vi "Line Configuration Dialog.vi"(8 "error in":errorcluster, 9 "engine configuration in":refnum<class "engine configuration.lvclass">, 10 "tag bus configurable plugin module configuration":refnum<class "JSON_RPC_Interface configuration.lvclass">, 11 "Line":T3) -> (0 "error out":errorcluster, 1 "success":bool, 2 "changed":bool, 3 "Mappings out":T2)   [LabVIEW 2018, in "JSON_RPC_Interface editor node.lvclass"]
doc: "A dialog for allowing a user to specify the values of a new line."
uses:
  JSON_RPC_Interface editor node.lvclass
  module/configuration/Line.ctl
  <vilib>/NI/Tag Bus Module Framework/channel/TBM channel.lvclass
  C:/Program Files (x86)/National Instruments/LabVIEW 2018/vi.lib/NI/Tag Bus/tag/tag descriptor.lvclass
  Mappings.ctl
  Map.ctl
  permissions.ctl
  <vilib>/NI/Module Execution Interface/Engine Configuration/engine configuration.lvclass
  module/configuration/JSON_RPC_Interface configuration.lvclass
  C:/Program Files (x86)/National Instruments/LabVIEW 2018/vi.lib/NI/Configuration Framework/serializable configuration/NISE_CEF_serializable configuration.lvclass
  <vilib>/NI/Tag Bus/tag/tag descriptor.lvclass/tag descriptor.ctl
  <vilib>/NI/Tag Bus Module Framework/channel/TBM channel.lvclass/TBM channel.ctl
  <vilib>/NI/Configuration Framework/serializable configuration/NISE_CEF_serializable configuration.lvclass/NISE_CEF_serializable configuration.ctl
  <vilib>/NI/Tag Bus Module Framework/channel/channel classification.ctl
  <vilib>/NI/Tag Bus Module Framework/channel/Read channel classification.vi
  <vilib>/NI/Tag Bus/tag/write tag name.vi
  <vilib>/NI/Tag Bus/tag/write data type.vi
  <vilib>/NI/Tag Bus Module Framework/channel/Write channel classification.vi
  <vilib>/NI/Configuration Framework/serializable configuration/Read UID.vi
  <vilib>/NI/Tag Bus/tag/read data type.vi
  <vilib>/Utility/LVClass/Get LV Class Name.vi
  <vilib>/NI/Configuration Framework/error generator/NISE_error generator.vi
  <vilib>/NI/Tag Bus/tag/tag descriptor.lvclass
  <vilib>/NI/DCAF UI Toolkit/Controls/DCAF UI Elements.lvlib
panel:
  out "errors":string
  in  "Access Type":T1
  in  "Tag":i32(listbox)
  in  "Data Type":i32(listbox)
  in  "cancel":bool
  in  "ok":bool
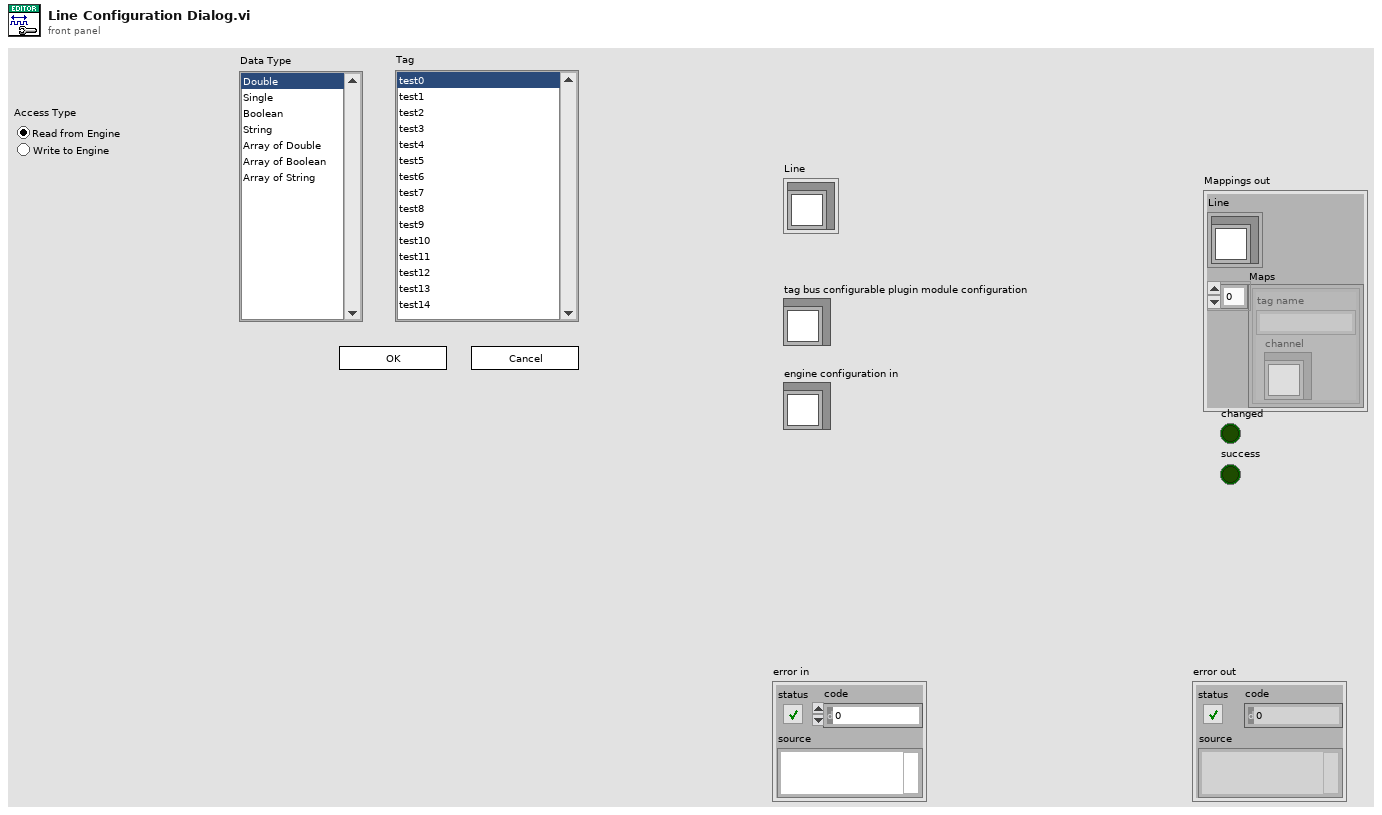
[diagram p1: front panel]
types:
  T1 = typedef "JSON_RPC_Interface editor node.lvclass/permissions.ctl" = enum32{"Read from Engine", "Write to Engine"}
  T2 = typedef "JSON_RPC_Interface editor node.lvclass/Mappings.ctl" = cluster{"Line":T3, "Maps":T4[]}
  T3 = typedef "JSON_RPC_Interface configuration.lvclass/Line.ctl" = cluster{"channel":refnum<class "TBM channel.lvclass">}
  T4 = typedef "JSON_RPC_Interface editor node.lvclass/Map.ctl" = cluster{"channel":refnum<class "TBM channel.lvclass">, "tag name":string}
  T5 = typedef "tag bus.lvlib/tag descriptor.lvclass/Data Type.ctl" = enum16{"Double", "Single", "I64", "I32", "I16", "I8", "U64", "U32", "U16", "U8", "Boolean", "String", "Array of Double", "Array of Single", "Array of I64", "Array of I32", "Array of I16", "Array of I8", "Array of U64", "Array of U32", "Array of U16", "Array of U8", "Array of Boolean", "Array of String"}
  T6 = typedef "TBM channel.lvclass/channel classification.ctl" = enum16{"input data", "output data", "processing parameter", "processing result"}
  T7 = enum8{"Enabled", "Disabled", "Disabled and Grayed Out"}
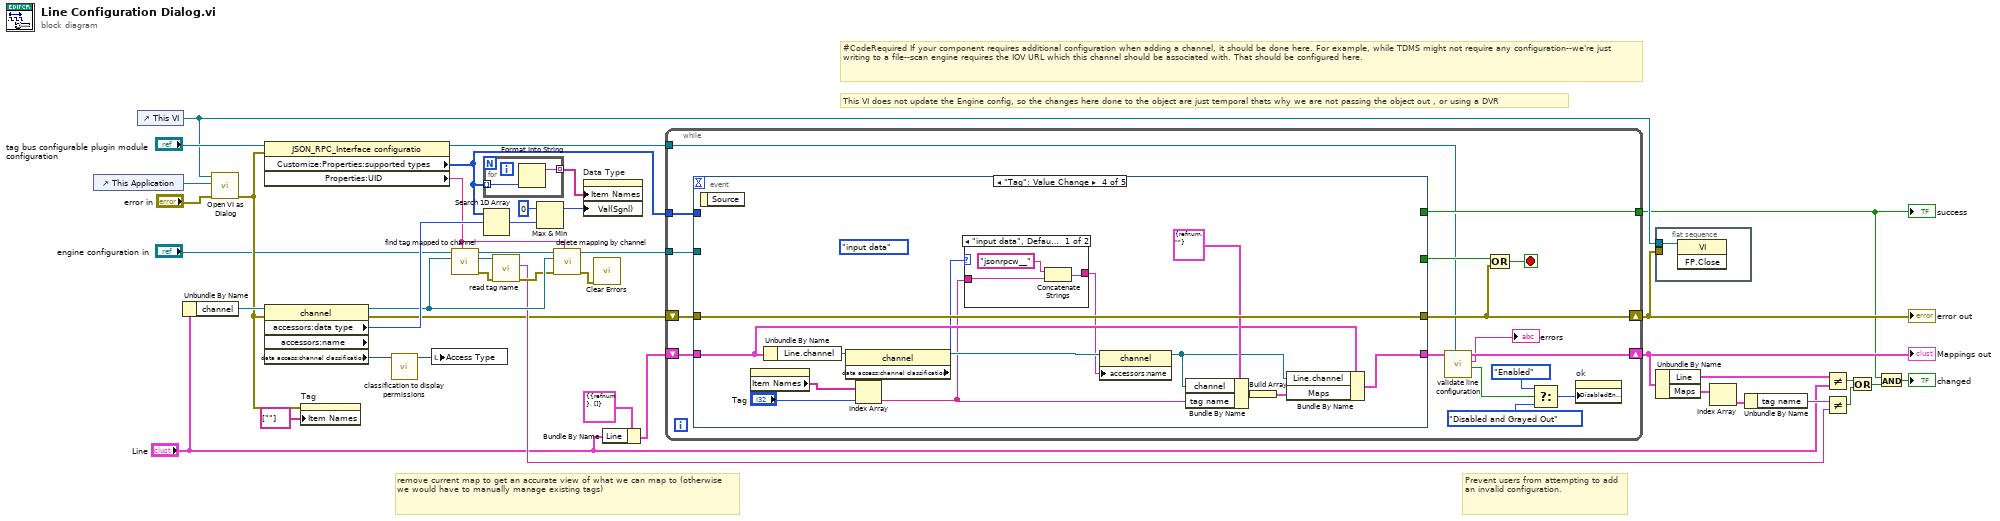
[diagram p0: block diagram]
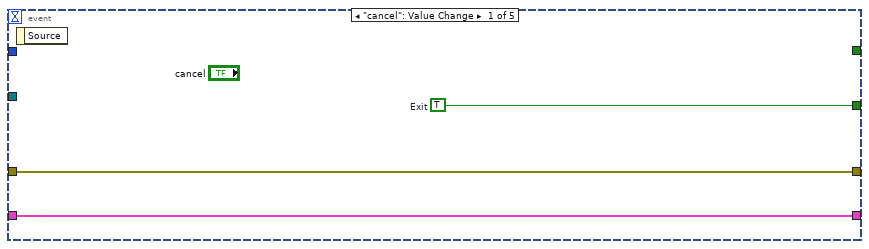
[diagram p2: hidden frame]
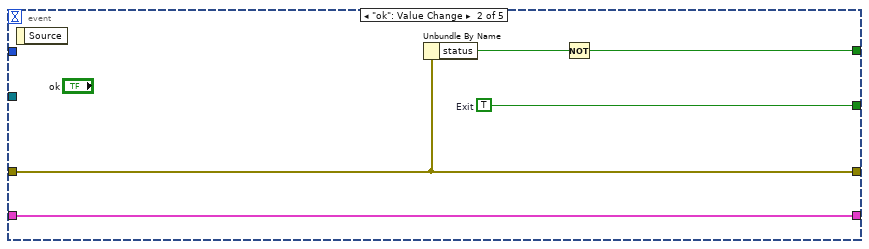
[diagram p3: hidden frame]
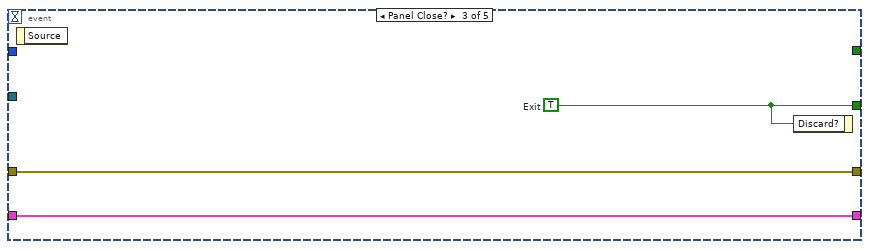
[diagram p4: hidden frame]
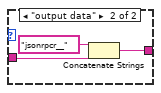
[diagram p5: hidden frame]
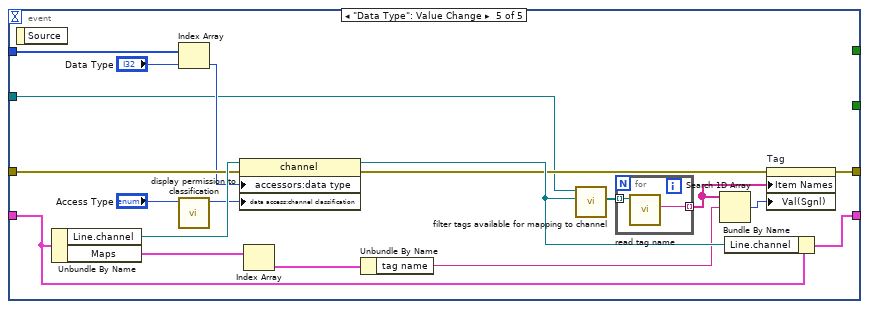
[diagram p6: hidden frame]
diagram:
  # "Prevent users from attempting to add an invalid configuration."
  # "This VI does not update the Engine config, so the changes here done to the object are just temporal thats why we are not passing the object out , or using a DVR"
  # "remove current map to get an accurate view of what we can map to (otherwise we would have to manually manage existing tags)"
  # "#CodeRequired If your component requires additional configuration when adding a channel, it should be done here. For example, while TDMS might not require any configuration--we're just writing to a file--scan engine requires the IOV URL which this channel should be associated with. That should be configured here."
  n1 = control-ref of="This Application"() -> (w30:refnum<vi>)
  n2 = control-ref of="This VI"() -> (w13:refnum<vi>)
  n3 = Unbundle By Name("Line") -> ("channel"=w40:refnum<class "TBM channel.lvclass">)
  n4 = call <vilib>:"Open VI as Dialog.vi"("error in (no error)"="error in", "This Application"=w30, "VI in"=w13) -> ("error out"=w28:errorcluster)  [unwired: 8 in]
  n5 = property class="JSON_RPC_Interface configuratio"(reference="tag bus configurable plugin module configuration", error in=w28) -> (reference out=w25:refnum<class "JSON_RPC_Interface configuration.lvclass">, "Customize:Properties:supported types"=w1:T5[], "Properties:UID"=w8:string)  [unwired: 1 out]
  n6 = property class="channel" props=["accessors:data type", "accessors:name", "data access:channel classification"](reference=w40, error in=w28) -> (reference out=w24:refnum<class "TBM channel.lvclass">, error out=w6:errorcluster, "accessors:data type"=w37:T5, "data access:channel classification"=w7:T6)  [unwired: 1 out]
  n7 = property on="Tag" class="LstBox (strict)"(error in=w28, "Item Names"=string[] [""]) -> ()  [unwired: 1 in, 2 out]
  n8 = call "classification to display permissions.vi"("channel classification"=w7) -> ("permissions"=w9:T1)  [unwired: 10 in]
  n9 = local write "Access Type"(w9) -> ()
  n10 = call <vilib>:"find tag mapped to channel.vi"("owner"=w8, "channel"=w24, "engine configuration in"="engine configuration in") -> ("error out"=w20:errorcluster, "tag"=w21:refnum<class "tag descriptor.lvclass">, "engine configuration out"=w26:refnum<class "engine configuration.lvclass">)  [unwired: 6 in]
  n11 = for {
    tunnel: w1 -> [w43] mode=indexing
    tunnel: [w42] -> w39 mode=indexing
    n12 = Format Into String(w43) -> (resulting string=w42:string)  [unwired: 3 in, 1 out]
  }
  n13 = Search 1D Array(1D array=w1, element=w37) -> (index of element=w23:i32)  [unwired: 1 in]
  n14 = call <vilib>:"read tag name.vi"("error in"=w20, "system tag in"=w21) -> ("error out"=w19:errorcluster, "name"=w12:string)  [unwired: 7 in, 1 out]
  n15 = Max & Min(x=0 ("f"), y=w23) -> (max(x,y)=w10:i32)  [unwired: 1 out]
  n16 = call <vilib>:"delete mapping by channel.vi"("owner ID"=w8, "error in"=w19, "channel"=w24, "engine configuration in"=w26) -> ("error out"=w36:errorcluster, "engine configuration out"=w41:refnum<class "engine configuration.lvclass">)  [unwired: 6 in]
  n17 = property on="Data Type" class="LstBox (strict)"("Item Names"=w39, "Val(Sgnl)"=w10) -> ()  [unwired: 2 in, 2 out]
  n18 = call <vilib>:"Clear Errors.vi"("error in (no error)"=w36) -> ()  [unwired: 5 in, 2 out]
  n19 = Bundle By Name(cluster=T2 {"Line"={"channel"=refnum}, "Maps"=[]} ("Mappings out"), "Line"="Line") -> (w33:T2)
  n20 = while {
    shift-right: [w51] -> w5
    shift-left: w6 -> [w58]
    tunnel: [w57] -> w4
    shift-right: [w52] -> w31
    shift-left: w33 -> [w54]
    tunnel: w41 -> [w59]
    tunnel: w25 -> [w46]
    tunnel: w1 -> [w45]
    stop <- w55 stop-if-true
    n21 = event shown="[3] \"Tag\": Value Change" {
      selector: _ -> [_ _ _ _ _]
      dyn-events: _ -> [_ _ _ _ _]
      timeout: _ -> [_ _ _ _ _]
      tunnel: w59 -> [_ _ _ _ w91]
      tunnel: w58 -> [w62 w65 w70 w84 w103]
      tunnel: [w62 w65 w70 w84 w98] -> w51
      tunnel: [_ w63 _ _ _] -> w57
      tunnel: [w60 w66 w68 _ _] -> w56
      tunnel: w54 -> [w61 w67 w69 w77 w92]
      tunnel: [w61 w67 w69 w78 w106] -> w53
      tunnel: w45 -> [_ _ _ _ w102]
      event "cancel": Value Change {
        w60 = TRUE  # Exit
        n22 = event-data() -> ()  [unwired: 1 in, 1 out]
      }
      event "ok": Value Change {
        w66 = TRUE  # Exit
        n23 = event-data() -> ()  [unwired: 1 in, 1 out]
        n24 = Unbundle By Name(w65) -> ("status"=w64:bool)
        n25 = Not(x=w64) -> (.not. x?=w63:bool)
      }
      event Panel Close? {
        w68 = TRUE  # Exit
        n26 = event-data() -> ()  [unwired: 1 in, 1 out]
        n27 = event-data("Discard?"=w68) -> ()  [unwired: 1 in, 1 out]
      }
      event "Tag": Value Change {
        (unwired) channel_classification."input data" ("channel classification")
        n28 = event-data() -> ()  [unwired: 1 in, 1 out]
        n29 = property on="Tag" class="LstBox (strict)"() -> ("Item Names"=w82:string[])  [unwired: 2 in, 2 out]
        n30 = Unbundle By Name(w77) -> ("Line.channel"=w76:refnum<class "TBM channel.lvclass">)
        n31 = property class="channel"(reference=w76) -> (reference out=w75:refnum<class "TBM channel.lvclass">, "data access:channel classification"=w74:T6)  [unwired: 1 in, 1 out]
        n32 = Index Array(array=w82, index="Tag") -> (element=w73:string)
        n33 = case shown="\"input data\", Default" w74 {
          tunnel: w73 -> [w85 w89]
          tunnel: [w87 w88] -> w72
          frame "input data", Default {
            n34 = Concatenate Strings("jsonrpcw__" ("string"), w85) -> (w87:string)
          }
          frame "output data" {
            n35 = Concatenate Strings("jsonrpcr__" ("string"), w89) -> (w88:string)
          }
        }
        n36 = property class="channel"(reference=w75, "accessors:name"=w72) -> (reference out=w71:refnum<class "TBM channel.lvclass">)  [unwired: 1 in, 1 out]
        n37 = Bundle By Name(cluster=T4 {"channel"=refnum, "tag name"=""} ("Map"), "channel"=w71, "tag name"=w73) -> (w80:T4)
        n38 = Build Array(w80) -> (w79:T4[])
        n39 = Bundle By Name(cluster=w77, "Line.channel"=w71, "Maps"=w79) -> (w78:T2)
      }
      event "Data Type": Value Change {
        n40 = event-data() -> ()  [unwired: 1 in, 1 out]
        n41 = Unbundle By Name(w92) -> ("Line.channel"=w109:refnum<class "TBM channel.lvclass">, "Maps"=w93:T4[])
        n42 = Index Array(array=w102, index="Data Type") -> (element=w100:T5)
        n43 = call "display permission to classification.vi"("display permissions"="Access Type") -> ("channel classification"=w108:T6)  [unwired: 10 in]
        n44 = property class="channel"(reference=w109, error in=w103, "accessors:data type"=w100, "data access:channel classification"=w108) -> (reference out=w107:refnum<class "TBM channel.lvclass">, error out=w99:errorcluster)
        n45 = Index Array(array=w93) -> (element=w95:T4)  [unwired: 1 in]
        n46 = Unbundle By Name(w95) -> ("tag name"=w94:string)
        n47 = call-dynamic "filter tags available for mapping to channel.vi"("channel to map to"=w107, "engine configuration in"=w91) -> ("filtered tags"=w105:refnum<class "tag descriptor.lvclass">[])  [unwired: 8 in, 1 out]
        n48 = for {
          tunnel: w105 -> [w111] mode=indexing
          tunnel: [w110] -> w97 mode=indexing
          n49 = call <vilib>:"read tag name.vi"("system tag in"=w111) -> ("name"=w110:string)  [unwired: 8 in, 2 out]
        }
        n50 = Search 1D Array(1D array=w97, element=w94) -> (index of element=w96:i32)  [unwired: 1 in]
        n51 = Bundle By Name(cluster=w92, "Line.channel"=w107) -> (w106:T2)
        n52 = property on="Tag" class="LstBox (strict)"(error in=w99, "Item Names"=w97, "Val(Sgnl)"=w96) -> (error out=w98:errorcluster)  [unwired: 1 in, 1 out]
      }
    }
    n53 = call "validate line configuration.vi"("Module Config"=w46, "Mappings in"=w53) -> ("valid?"=w50:bool, "errors"=→"errors":string, "Mappings out"=w52:T2)  [unwired: 7 in]
    n54 = Compound Arithmetic op=OR(w56, w51) -> (w55:bool)
    n55 = Select(t=T7."Enabled" ("Disabled"), s=w50, f=T7."Disabled and Grayed Out") -> (s? t:f=w47:T7)
    n56 = property on="ok" class="Bool"("DisabledEnum"=w47) -> ()  [unwired: 2 in, 2 out]
  }
  "error out" <- w5
  "success" <- w4
  "Mappings out" <- w31
  n57 = flat-sequence {
    tunnel: w5 -> [_]
    tunnel: w13 -> [w112]
    frame #0 {
      n58 = invoke class="VI" method="FP.Close"(reference=w112) -> ()  [unwired: 2 in, 3 out]
    }
  }
  n59 = Unbundle By Name(w31) -> ("Line"=w32:T3, "Maps"=w18:T4[])
  n60 = Index Array(array=w18) -> (element=w17:T4)  [unwired: 1 in]
  n61 = Unbundle By Name(w17) -> ("tag name"=w16:string)
  n62 = Not Equal?(x=w32, y="Line") -> (x != y?=w14:bool)
  n63 = Not Equal?(x=w16, y=w12) -> (x != y?=w15:bool)
  n64 = Or(x=w14, y=w15) -> (x .or. y?=w3:bool)
  n65 = And(x=w4, y=w3) -> (x .and. y?=→"changed":bool)
